vi "stage_setposition.vi"(8 "error in (no error)":errorcluster, 9 "speeds":T1={"speedx"=4.0, "speedy"=4.0, "speedz"=4.0} {"speedx" min=0 max=4; "speedy" min=0 max=4; "speedz" min=0 max=4}, 10 "Position in[µm]":T2={"xposition[µm]"=100.0, "yposition[µm]"=200.0, "zposition[µm]"=200.0} {"xposition[µm]" min=100 max=3900; "yposition[µm]" min=200 max=3800; "zposition[µm]" min=200 max=3800}, 11 "Stage reference in":T3) -> (0 "error out":errorcluster, 3 "Stage reference out":T3)   [LabVIEW 2018]
uses:
  stage_reference_type.ctl
  <userlib>/stepper/velocity settings.ctl
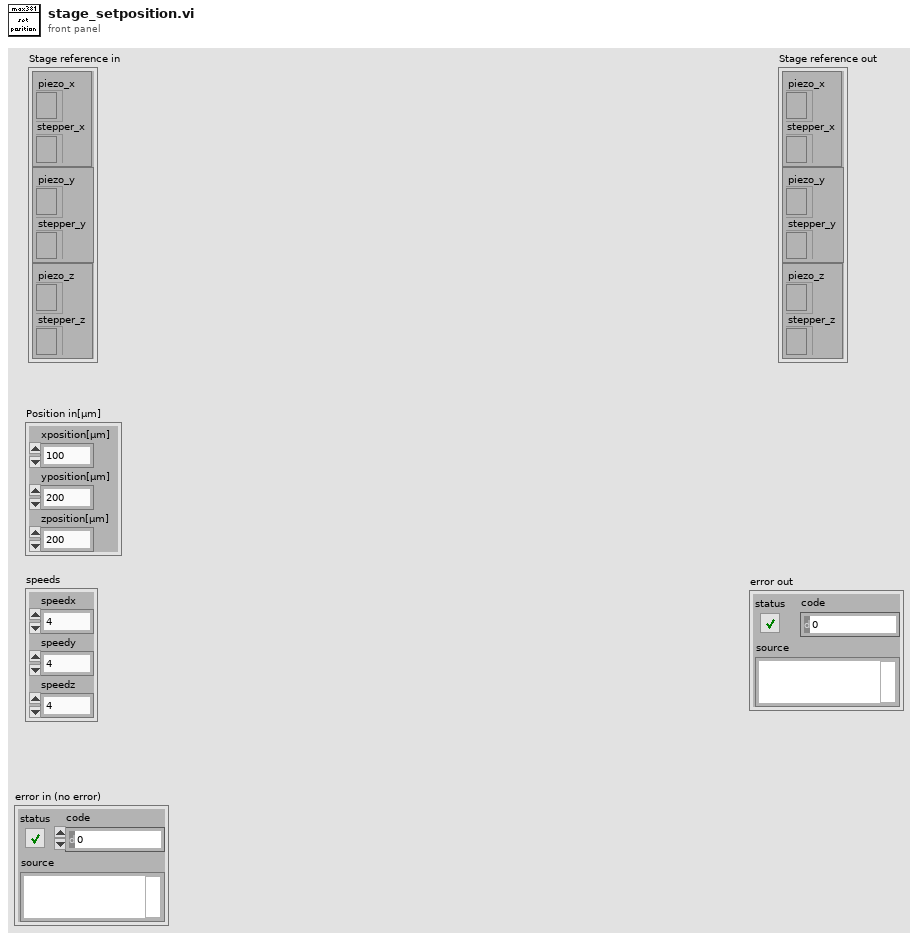
[diagram p1: front panel]
types:
  T1 = cluster{"speedx":sgl, "speedy":sgl, "speedz":sgl}
  T2 = cluster{"xposition[µm]":sgl, "yposition[µm]":sgl, "zposition[µm]":sgl}
  T3 = typedef "stage_reference_type.ctl" = cluster{cluster{"piezo_x":refnum<k7>, "stepper_x":refnum<k7>}, cluster{"piezo_y":refnum<k7>, "stepper_y":refnum<k7>}, cluster{"piezo_z":refnum<k7>, "stepper_z":refnum<k7>}}
  T4 = typedef "velocity settings.ctl" = cluster{"pfMinVel":sgl, "pfAccn":sgl, "pfMaxVel":sgl}
  T5 = cluster{"piezo_x":refnum<k7>, "stepper_x":refnum<k7>}
  T6 = cluster{"piezo_y":refnum<k7>, "stepper_y":refnum<k7>}
  T7 = cluster{"piezo_z":refnum<k7>, "stepper_z":refnum<k7>}
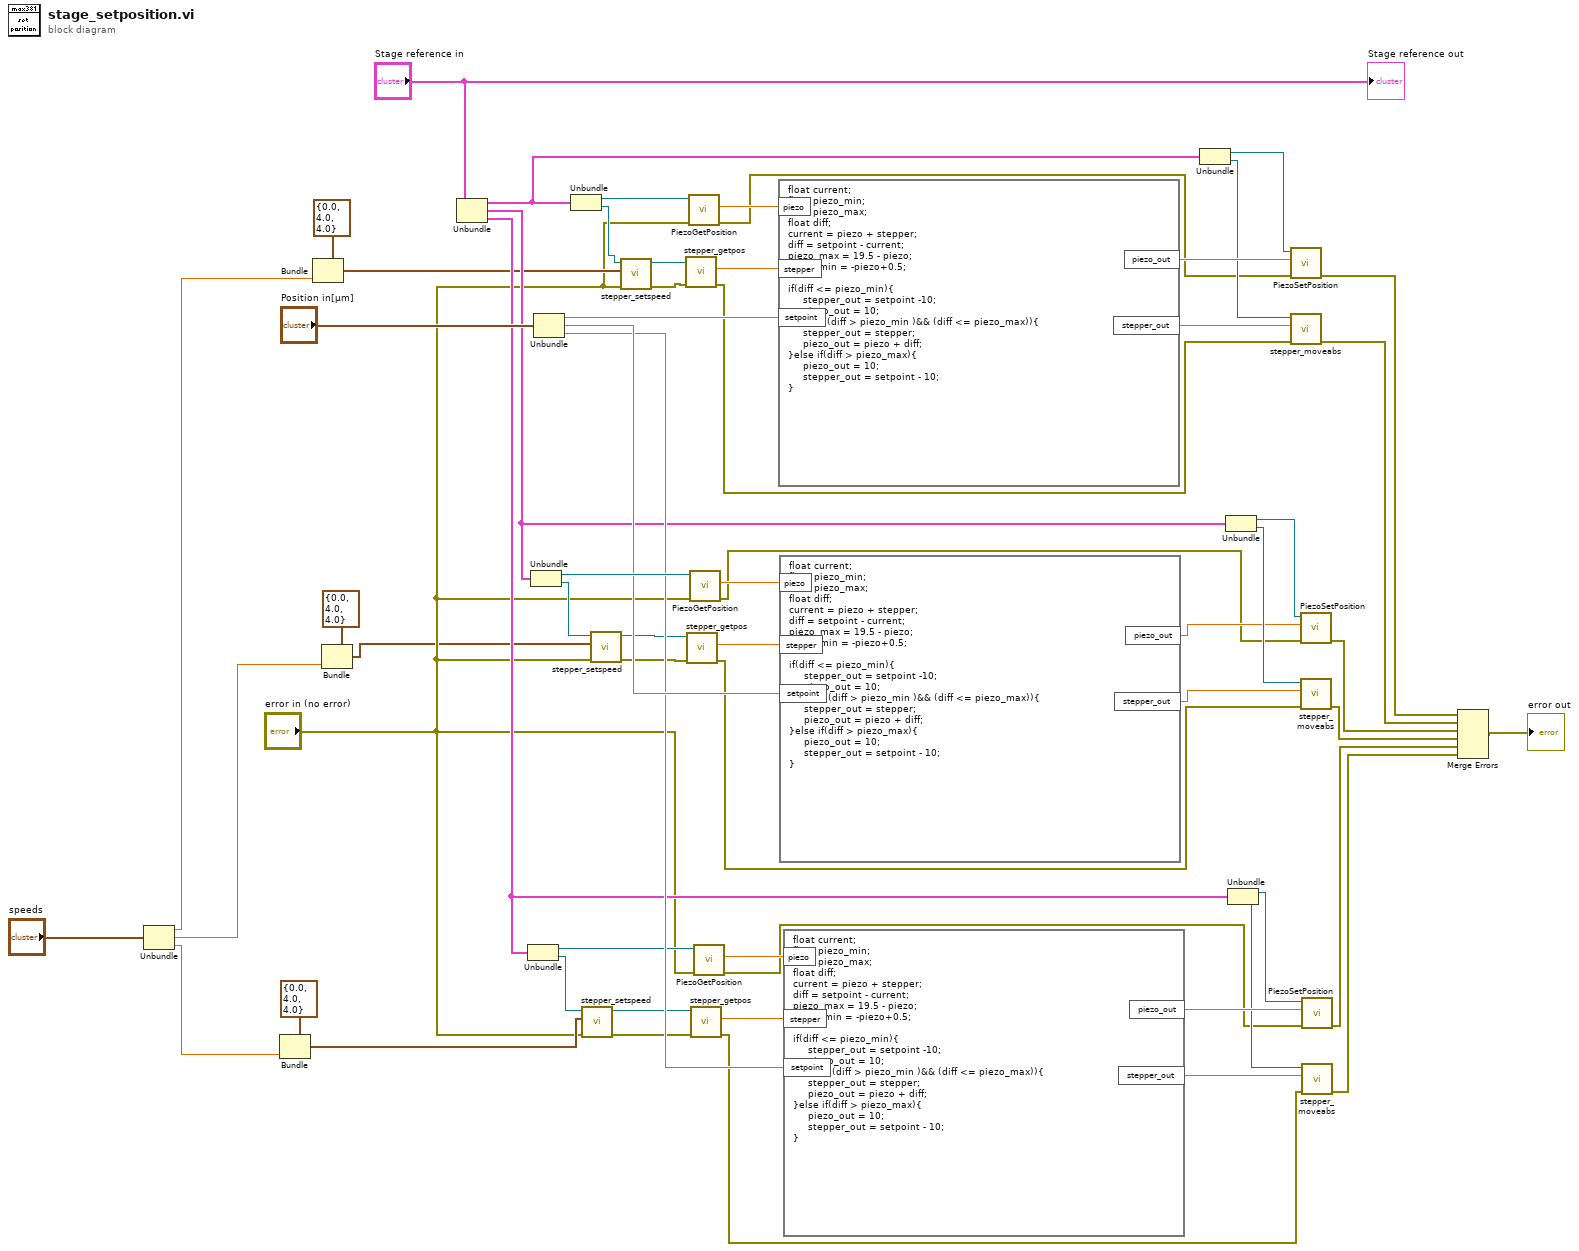
[diagram p0: block diagram]
diagram:
  n1 = Unbundle("speeds") -> ("speedx"=w6:sgl, "speedy"=w7:sgl, "speedz"=w8:sgl)
  n2 = Bundle(cluster=T4 {"pfMinVel"=0.0, "pfAccn"=4.0, "pfMaxVel"=4.0} ("velocity parameters in"), "pfMaxVel"=w8) -> (w4:T4)  [unwired: 2 in]
  n3 = Bundle(cluster=T4 {"pfMinVel"=0.0, "pfAccn"=4.0, "pfMaxVel"=4.0} ("velocity parameters in"), "pfMaxVel"=w6) -> (w5:T4)  [unwired: 2 in]
  n4 = Bundle(cluster=T4 {"pfMinVel"=0.0, "pfAccn"=4.0, "pfMaxVel"=4.0} ("velocity parameters in"), "pfMaxVel"=w7) -> (w1:T4)  [unwired: 2 in]
  n5 = Unbundle("Stage reference in") -> (w46:T5, w47:T6, w48:T7)
  n6 = Unbundle(w48) -> ("piezo_z"=w49:refnum<k7>, "stepper_z"=w14:refnum<k7>)
  n7 = Unbundle(w47) -> ("piezo_y"=w57:refnum<k7>, "stepper_y"=w17:refnum<k7>)
  n8 = Unbundle("Position in[µm]") -> ("xposition[µm]"=w58:sgl, "yposition[µm]"=w51:sgl, "zposition[µm]"=w50:sgl)
  n9 = Unbundle(w46) -> ("piezo_x"=w61:refnum<k7>, "stepper_x"=w20:refnum<k7>)
  n10 = call <userlib>:"stepper_setspeed.vi"("error in (no error)"="error in (no error)", "velocity parameters in"=w4, "reference"=w14) -> ("error out"=w3:errorcluster, "reference out"=w13:refnum<k7>)  [unwired: 6 in, 1 out]
  n11 = call <userlib>:"stepper_setspeed.vi"("error in (no error)"="error in (no error)", "velocity parameters in"=w1, "reference"=w17) -> ("error out"=w16:errorcluster, "reference out"=w18:refnum<k7>)  [unwired: 6 in, 1 out]
  n12 = call <userlib>:"stepper_setspeed.vi"("error in (no error)"="error in (no error)", "velocity parameters in"=w5, "reference"=w20) -> ("error out"=w15:errorcluster, "reference out"=w19:refnum<k7>)  [unwired: 6 in, 1 out]
  n13 = call <userlib>:"stepper_getpos.vi"("error in (no error)"=w15, "reference"=w19) -> ("error out"=w31:errorcluster, "pfPosition[µm]"=w59:sgl)  [unwired: 7 in, 1 out]
  n14 = call <userlib>:"stepper_getpos.vi"("error in (no error)"=w16, "reference"=w18) -> ("error out"=w28:errorcluster, "pfPosition[µm]"=w55:sgl)  [unwired: 7 in, 1 out]
  n15 = call <userlib>:"PiezoGetPosition.vi"("error in (no error)"="error in (no error)", "reference"=w61) -> ("error out"=w32:errorcluster, "Position"=w60:sgl)  [unwired: 3 in, 1 out]
  n16 = call <userlib>:"PiezoGetPosition.vi"("error in (no error)"="error in (no error)", "reference"=w57) -> ("error out"=w29:errorcluster, "Position"=w56:sgl)  [unwired: 3 in, 1 out]
  n17 = call <userlib>:"stepper_getpos.vi"("error in (no error)"=w3, "reference"=w13) -> ("error out"=w24:errorcluster, "pfPosition[µm]"=w53:sgl)  [unwired: 7 in, 1 out]
  n18 = call <userlib>:"PiezoGetPosition.vi"("error in (no error)"="error in (no error)", "reference"=w49) -> ("error out"=w25:errorcluster, "Position"=w54:sgl)  [unwired: 3 in, 1 out]
  n19 = formula code="float current;\nfloat piezo_min;\nfloat piezo_max;\nfloat diff;\ncurrent = piezo + stepper;\ndiff = setpoint - current;\npiezo_max = 19.5 - piezo;\npiezo_min = -piezo+0.5;\n\nif(diff <= piezo_min){\n     stepper_out = setpoint -10;\n     piezo_out = 10;\n}else if((diff > piezo_min )&& (diff <= piezo_max)){\n     stepper_out = stepper;\n     piezo_out = piezo + diff;\n}else if(diff > piezo_max){\n     piezo_out = 10;\n     stepper_out = setpoint - 10;\n}"("piezo"=w60, "stepper"=w59, "setpoint"=w58) -> ("piezo_out"=w44:dbl, "stepper_out"=w43:dbl)
  n20 = formula code="float current;\nfloat piezo_min;\nfloat piezo_max;\nfloat diff;\ncurrent = piezo + stepper;\ndiff = setpoint - current;\npiezo_max = 19.5 - piezo;\npiezo_min = -piezo+0.5;\n\nif(diff <= piezo_min){\n     stepper_out = setpoint -10;\n     piezo_out = 10;\n}else if((diff > piezo_min )&& (diff <= piezo_max)){\n     stepper_out = stepper;\n     piezo_out = piezo + diff;\n}else if(diff > piezo_max){\n     piezo_out = 10;\n     stepper_out = setpoint - 10;\n}"("piezo"=w56, "stepper"=w55, "setpoint"=w51) -> ("piezo_out"=w35:dbl, "stepper_out"=w34:dbl)
  n21 = formula code="float current;\nfloat piezo_min;\nfloat piezo_max;\nfloat diff;\ncurrent = piezo + stepper;\ndiff = setpoint - current;\npiezo_max = 19.5 - piezo;\npiezo_min = -piezo+0.5;\n\nif(diff <= piezo_min){\n     stepper_out = setpoint -10;\n     piezo_out = 10;\n}else if((diff > piezo_min )&& (diff <= piezo_max)){\n     stepper_out = stepper;\n     piezo_out = piezo + diff;\n}else if(diff > piezo_max){\n     piezo_out = 10;\n     stepper_out = setpoint - 10;\n}"("piezo"=w54, "stepper"=w53, "setpoint"=w50) -> ("piezo_out"=w41:dbl, "stepper_out"=w40:dbl)
  n22 = Unbundle(w46) -> ("piezo_x"=w45:refnum<k7>, "stepper_x"=w42:refnum<k7>)
  n23 = Unbundle(w47) -> ("piezo_y"=w36:refnum<k7>, "stepper_y"=w37:refnum<k7>)
  n24 = Unbundle(w48) -> ("piezo_z"=w39:refnum<k7>, "stepper_z"=w38:refnum<k7>)
  n25 = call <userlib>:"PiezoSetPosition.vi"("error in (no error)"=w32, "pos in"=w44, "reference"=w45) -> ("error out"=w33:errorcluster)  [unwired: 3 in, 1 out]
  n26 = call <userlib>:"stepper_moveabs.vi"("error in (no error)"=w31, "fAbsPos[µm]"=w43, "reference"=w42) -> ("error out"=w30:errorcluster)  [unwired: 7 in, 1 out]
  n27 = call <userlib>:"PiezoSetPosition.vi"("error in (no error)"=w29, "pos in"=w35, "reference"=w36) -> ("error out"=w26:errorcluster)  [unwired: 3 in, 1 out]
  n28 = call <userlib>:"stepper_moveabs.vi"("error in (no error)"=w28, "fAbsPos[µm]"=w34, "reference"=w37) -> ("error out"=w27:errorcluster)  [unwired: 7 in, 1 out]
  n29 = call <userlib>:"PiezoSetPosition.vi"("error in (no error)"=w25, "pos in"=w41, "reference"=w39) -> ("error out"=w23:errorcluster)  [unwired: 3 in, 1 out]
  n30 = call <userlib>:"stepper_moveabs.vi"("error in (no error)"=w24, "fAbsPos[µm]"=w40, "reference"=w38) -> ("error out"=w22:errorcluster)  [unwired: 7 in, 1 out]
  n31 = Merge Errors(w33, w30, w26, w27, w23, w22) -> (→"error out":errorcluster)
  "Stage reference out" <- "Stage reference in"
